vi "ready.vi"(8 "error in (no error)":errorcluster, 11 "control refs in":T1) -> (0 "error out":errorcluster, 3 "control refs out":T1)   [LabVIEW 2010]
uses:
  type_definitions/clusters/controls_refs.ctl
  type_definitions/enumerations/main_control_types.ctl
  components/ImagingMode/GenericImagingMode/GenericImagingMode/GenericImagingMode.lvclass
  components/ImagingMode/GenericImagingMode/GenericImagingMode/trigger_enum.ctl
  global_variables.vi
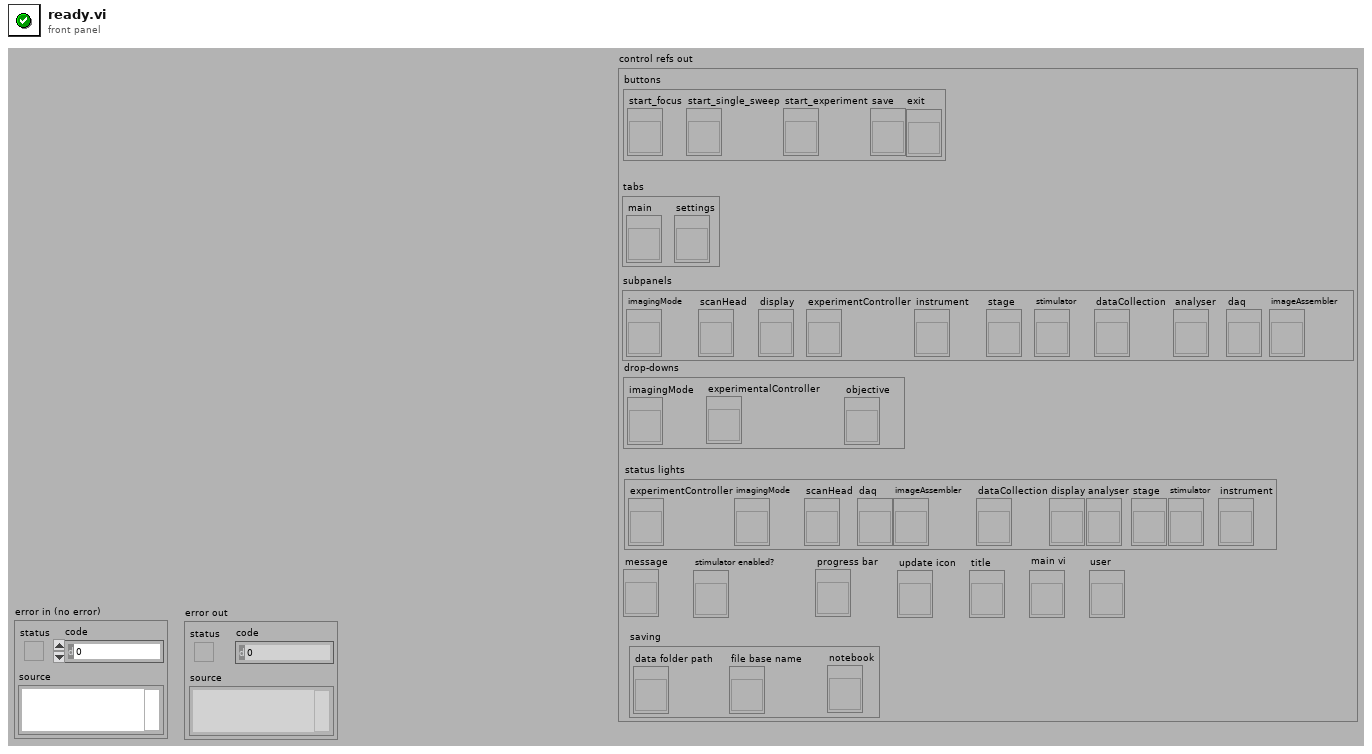
[diagram p1: front panel]
types:
  T1 = typedef "controls_refs.ctl" = cluster{"buttons":cluster{"start_focus":refnum<vi>, "start_single_sweep":refnum<vi>, "start_experiment":refnum<vi>, "save":refnum<vi>, "exit":refnum<vi>}, "tabs":cluster{"main":refnum<vi>, "settings":refnum<vi>}, "subpanels":cluster{"imagingMode":refnum<vi>, "scanHead":refnum<vi>, "display":refnum<vi>, "experimentController":refnum<vi>, "instrument":refnum<vi>, "stage":refnum<vi>, "stimulator":refnum<vi>, "dataCollection":refnum<vi>, "analyser":refnum<vi>, "daq":refnum<vi>, "imageAssembler":refnum<vi>}, "drop-downs":cluster{"imagingMode":refnum<vi>, "experimentalController":refnum<vi>, "objective":refnum<vi>}, "status lights":cluster{"experimentController":refnum<vi>, "imagingMode":refnum<vi>, "scanHead":refnum<vi>, "daq":refnum<vi>, "imageAssembler":refnum<vi>, "dataCollection":refnum<vi>, "display":refnum<vi>, "analyser":refnum<vi>, "stage":refnum<vi>, "stimulator":refnum<vi>, "instrument":refnum<vi>}, "message":refnum<vi>, "stimulator enabled?":refnum<vi>, "saving":cluster{"data folder path":refnum<vi>, "file base name":refnum<vi>, "notebook":refnum<vi>}, "progress bar":refnum<vi>, "update icon":refnum<vi>, "title":refnum<vi>, "main vi":refnum<vi>, "user":refnum<vi>}
  T2 = enum8{"Enabled", "Disabled", "Disabled and Grayed Out"}
  T3 = typedef "GenericImagingMode.lvclass/trigger_enum.ctl" = enum16{"NULL", "proceed"}
  T4 = typedef "main_control_types.ctl" = enum16{"scan start button", "experimentController subpanel", "imagingMode subpanel", "scanHead subpanel", "dataCollection subpanel", "display subpanel", "analyser subpanel", "stimulator subpanel", "run mode drop-down", "imagingMode drop-down", "experimentController drop-down", "objective drop-down", "exit button"}
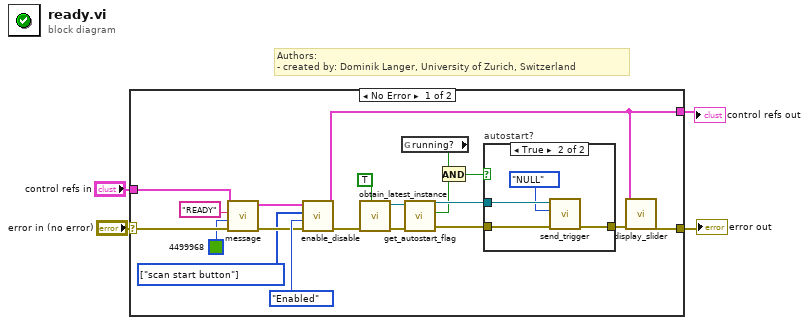
[diagram p0: block diagram]
diagram:
  # "Authors: \n- created by: Dominik Langer, University of Zurich, Switzerland"
  n1 = case shown="No Error" "error in (no error)" {
    selector: "error in (no error)" -> [w16 w31]
    tunnel: [w12 w31] -> w3
    tunnel: "control refs in" -> [w7 w30]
    tunnel: [w6 w30] -> w1
    frame No Error {
      w5 = T4[] [enum."scan start button"] items=["scan start button", "experimentController subpanel", "imagingMode subpanel", "scanHead subpanel", "dataCollection subpanel", "display subpanel", "analyser subpanel", "stimulator subpanel", "run mode drop-down", "imagingMode drop-down", "experimentController drop-down", "objective drop-down", "exit button"]
      n2 = call "message.vi"("error in (no error)"=w16, "BG slider"=u32 4499968, "text"="READY", "control references in"=w7) -> ("error out"=w10:errorcluster, "control references out"=w8:T1)  [unwired: 3 in, 3 out]
      n3 = call "enable_disable.vi"("error in (no error)"=w10, "state"=T2."Enabled", "controls"=w5, "control references in"=w8) -> ("error out"=w9:errorcluster, "control references out"=w6:T1)  [unwired: 6 in]
      n4 = call "obtain_latest_instance.vi"("quick, but maybe outdated?"=TRUE, "error in (no error)"=w9) -> ("error out"=w22:errorcluster, "GenericScanMode out"=w23:refnum<class "GenericImagingMode.lvclass">)  [unwired: 8 in]
      n5 = global read "global_variables.vi" "running?"() -> (w19:bool)
      n6 = call-dynamic "get_autostart_flag.vi"("error in (no error)"=w22, "GenericScanMode in"=w23) -> ("error out"=w21:errorcluster, "autostart?"=w18:bool, "GenericScanMode out"=w20:refnum<class "GenericImagingMode.lvclass">)  [unwired: 7 in]
      n7 = And(x=w19, y=w18) -> (x .and. y?=w17:bool)
      n8 = case "autostart?" shown="True" w17 {
        tunnel: w21 -> [w25 w29]
        tunnel: w20 -> [_ w28]
        tunnel: [w25 w26] -> w13
        frame False {
        }
        frame True {
          n9 = call-dynamic "send_trigger.vi"("error in (no error)"=w29, "message"=trigger_enum."NULL", "GenericScanMode in"=w28) -> ("error out"=w26:errorcluster)  [unwired: 7 in, 1 out]
        }
      }
      n10 = call "display_slider.vi"("error in"=w13, "cluster refs in"=w6) -> ("error out"=w12:errorcluster)  [unwired: 9 in]
    }
    frame Error {
    }
  }
  "error out" <- w3
  "control refs out" <- w1
